vi "Write DAQmx active_nonactive.vi"(8 "error in (no error)":errorcluster, 10 "DAQmx active/nonactive":bool, 11 "Control in":refnum<class "Control.lvclass">) -> (0 "error out":errorcluster, 3 "Control out":refnum<class "Control.lvclass">)   [LabVIEW 2015, in "Control.lvclass"]
uses:
  Control.lvclass
  Control.lvclass/Control.ctl
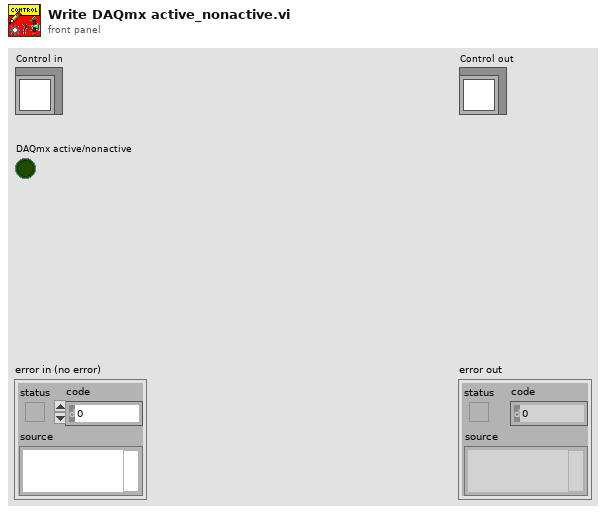
[diagram p1: front panel]
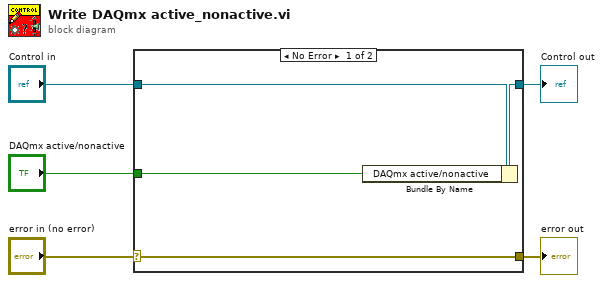
[diagram p0: block diagram]
diagram:
  n1 = case shown="No Error" "error in (no error)" {
    selector: "error in (no error)" -> [w9 w10]
    tunnel: [w9 w10] -> w4
    tunnel: [w7 w11] -> w2
    tunnel: "Control in" -> [w8 w11]
    tunnel: "DAQmx active/nonactive" -> [w6 _]
    frame No Error {
      n2 = Bundle By Name(cluster=w8, "DAQmx active/nonactive"=w6) -> (w7:refnum<class "Control.lvclass">)
    }
    frame Error {
    }
  }
  "error out" <- w4
  "Control out" <- w2
